vi "TimeLmtDialog.vi"(8 "颜色盒":u32(colorbox), 9 "time(s)":i32=5, 10 "Infoin":string="在这里填写显示的信息内容", 11 "title":string="提示信息") -> ()   [LabVIEW 2016]
panel:
  in  "ok":bool
  out "info":string
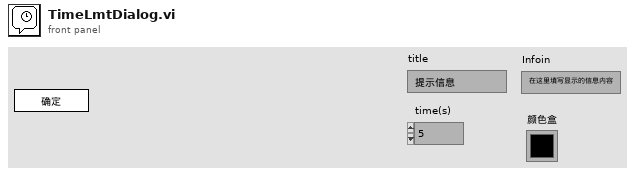
[diagram p1: front panel]
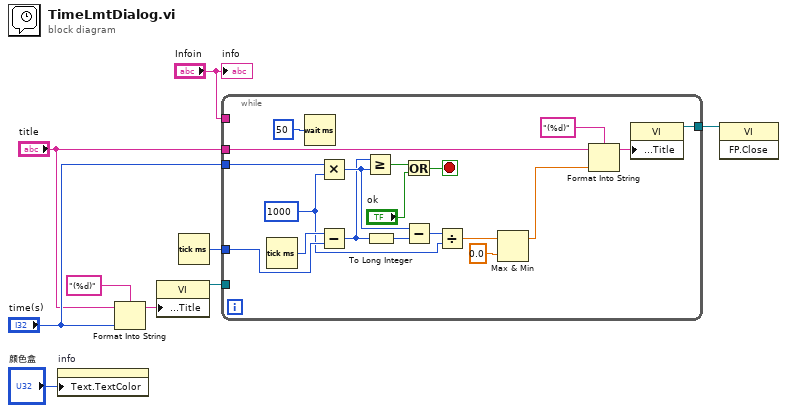
[diagram p0: block diagram]
diagram:
  n1 = property on="info" class="Str"("Text.TextColor"="颜色盒") -> ()  [unwired: 2 in, 2 out]
  n2 = Format Into String(format string="(%d)" ("格式字符串"), initial string="title", "time(s)") -> (resulting string=w5:string)  [unwired: 1 in, 1 out]
  n3 = property class="VI"("Front Panel.Title"=w5) -> (reference out=w8:refnum<vi>)  [unwired: 2 in, 1 out]
  n4 = Tick Count (ms)() -> (millisecond timer value=w3:u32)
  n5 = while {
    tunnel: "Infoin" -> [_]
    tunnel: "time(s)" -> [w25]
    tunnel: w8 -> [_]
    tunnel: "title" -> [w17]
    tunnel: w3 -> [w26]
    tunnel: [w10] -> w2
    stop <- w22 stop-if-true
    w18 = 1000 ("y")
    n6 = Tick Count (ms)() -> (millisecond timer value=w27:u32)
    n7 = Wait (ms)(milliseconds to wait=u32 50 ("等待时间（毫秒）")) -> ()  [unwired: 1 out]
    n8 = Multiply(x=w25, y=w18) -> (x*y=w21:i32)
    n9 = Subtract(x=w27, y=w26) -> (x-y=w20:u32)
    n10 = Greater Or Equal?(x=w20, y=w21) -> (x >= y?=w23:bool)
    n11 = To Long Integer(number=w20) -> (32bit integer=w11:i32)
    n12 = Or(x=w23, y="ok") -> (x .or. y?=w22:bool)
    n13 = Subtract(x=w21, y=w11) -> (x-y=w19:i32)
    n14 = Divide(x=w19, y=w18) -> (x/y=w14:dbl)
    n15 = Max & Min(x=w14, y=0.0) -> (max(x,y)=w12:dbl)  [unwired: 1 out]
    n16 = Format Into String(format string="(%d)" ("格式字符串"), initial string=w17, w12) -> (resulting string=w15:string)  [unwired: 1 in, 1 out]
    n17 = property class="VI"("Front Panel.Title"=w15) -> (reference out=w10:refnum<vi>)  [unwired: 2 in, 1 out]
  }
  n18 = invoke class="VI" method="FP.Close"(reference=w2) -> ()  [unwired: 2 in, 3 out]
  "info" <- "Infoin"
